vi "hpcnc try reset status.vi"(8 "error in (no error)":errorcluster, 11 "VISA Refnum in":refnum<visa-resource-name>) -> ()   [LabVIEW 2014]
uses:
  HPCNC.lvlib
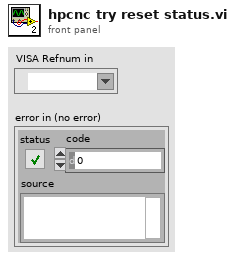
[diagram p1: front panel]
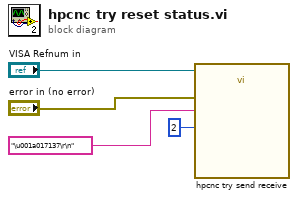
[diagram p0: block diagram]
diagram:
  n1 = call "hpcnc try send receive.vi"("error in (no error)"="error in (no error)", "Max try number"=2, "Send package"="\u001a017137\r\n", "VISA Refnum in"="VISA Refnum in") -> ()  [unwired: 4 in, 4 out]
